vi "foucault control panel.vi"() -> ()   [LabVIEW 2017]
uses:
  typedefs/gain setting.ctl
  typedefs/commandType.ctl
  <vilib>/Analysis/baseanly.llb/Mean (DBL).vi
  popup panels/control panel globals.vi
  <vilib>/Analysis/NI_AALBase.lvlib
panel:
  out "orbit for display":T1 {"height" format="%.1f"; "y offset" format="%.1f"; "x offset" format="%.1f"; "mag  tilt (d)" format="%.1f"; "ax angle (d)" format="%.1f"; "minor axis" format="%.1f"; "maj axis" format="%.1f"}
  out "working magnetomters":bool[](array[boolean])
  out "pulse energy (uJ)":dbl
  out "pulse charge (mC)":sgl
  in  "pulse coil":bool
  in  "zero voltage":bool
  out "predicted precession (deg/hr)":dbl format="%.1f"
  out "minor axis (mm)":dbl format="%.1f"
  in  "bob mass (g)":dbl=550.0
  out "amplitude (mm)":dbl format="%.1f"
  in  "take snapshot":bool
  in  "reset auto coil on pico":bool
  in  "zero field":bool
  in  "num readings\n to average":i32=100 min=1 step=1
  out "gain":dbl
  in  "visible":bool[](array[boolean])=[FALSE, FALSE, FALSE, FALSE, FALSE, FALSE]
  out "pop-up panels":string[](array[string])
  in  "autoscale mag":bool=TRUE
  out "re-synch":bool
  in  "toggle led automatically?":enum16{"NEVER", "WITH COIL", "HALF CYCLE"}(ring)
  out "mag field":cluster{"x":dbl, "y":dbl, "z":dbl}
  out "orbit is":enum16{"clockwise", "counterclockwise"}(ring)
  in  "Freeze Display":bool
  in  "mag type":enum16{"absolute", "relative", "positional"}(ring)
  out "L (m)":dbl
  in  "Display type":enum16{"rolling", "triggered"}(ring)
  in  "Trigger direction":enum16{"falling edge", "rising edge"}(ring)=enum."rising edge"
  out "firmware version":dbl
  in  "auto coil":bool
  in  "pulse duration (ms)":dbl=5.0 format="%#_6f"
  in  "pulse phase (deg)":dbl=40.0 format="%#_6p"
  in  "Gain setting":T2=enum."16.25"
  in  "LED level":u8(slide) scale=0.0..255.0
  in  "manual coil activation":bool
  out "Period":dbl
  in  "hysteresis":dbl=0.05 format="%.3f"
  out "magnet":cluster{dbl[], "Best Linear Fit":dbl[]}[](graph)
  in  "time range (s)":dbl=3.0 format="%#_13g"
  out "voltage":cluster{dbl[], dbl[]}[](graph)
  out "error out":errorcluster
  in  "stop program":bool
  out "VISA resource name":refnum<visa-resource-name>
  # "Update date: 9/28/2022\n(Lab 2 - Fall 2022)"
types:
  T1 = cluster{"maj axis":dbl, "minor axis":dbl, "ax angle (d)":dbl, "mag  tilt (d)":dbl, "x offset":dbl, "y offset":dbl, "height ":dbl}
  T2 = typedef "gain setting.ctl" = enum16{"7.87", "16.25", "30.5", "58.7", "120.6", "238.6", "477.3", "954.6"}
  T3 = typedef "queue cluster.ctl" = cluster{"voltage":T4, "coil":T4, "mag":refnum<queue>, "accel":T4, "crossing":T4, "orbit fit":refnum<queue>, "pulse":T4, "mag0":T4, "fitLocation":refnum<queue>}
  T4 = typedef "reading queue.ctl" = refnum<queue>
  T5 = typedef "reading.ctl" = cluster{"reading type":T6, "time":fxp<+,48,48>, "x":sgl, "y":sgl, "z":sgl, "XSUM":u8}
  T6 = typedef "readingType.ctl" = enum8{"SYNC", "DETVAL", "COILI", "MAGVEC", "ACCVEC", "CROSSING", "MAGVEC0", "MAGVEC1", "MAGVEC2", "MAGVEC3", "MAGVEC4", "MAGVEC5", "MAGVEC6", "MAGVEC7"}
  T7 = typedef "crossing stats.ctl" = cluster{"recent crossing":dbl, "prev crossing":dbl, "crossing-2":dbl, "number of crossings":i32, "period":dbl, "new crossing":bool, "new odd crossing":bool, "slope":dbl}
  T8 = cluster{"maj axis":dbl, "minor axis":dbl, "axis angle (deg)":dbl, "magnet tilt (deg)":dbl, "x offset":dbl, "y offset":dbl, "height above sensor":dbl}
  T9 = enum16{"absolute", "relative", "positional", "position only"}
  T10 = cluster{"pulse energy (uJ)":sgl, "pulse phase":dbl, "v":dbl, "I dt":dbl, "pulse time":dbl, "timing error":dbl}
  T11 = enum32{"Invalid", "Standard", "Closed", "Hidden", "Minimized", "Maximized"}
  T12 = cluster{" xrange":cluster{dbl, dbl}, "yrange":cluster{dbl, dbl}}
  T13 = cluster{"Best Linear Fit":dbl[], "Best Linear Fit":dbl[]}[]
  T14 = typedef "commandType.ctl" = enum16{"G - set gain", "C - activate coil", "D - deactivate coil", "L - set LED", "A - set AUTO", "V - set verbose", "T - set transmission", "R - get version", "Z - zero accelerometer", "F - set auto-flash led", "X - synchronize serial", "Q - reset queues and timers", "S - save configuration"}
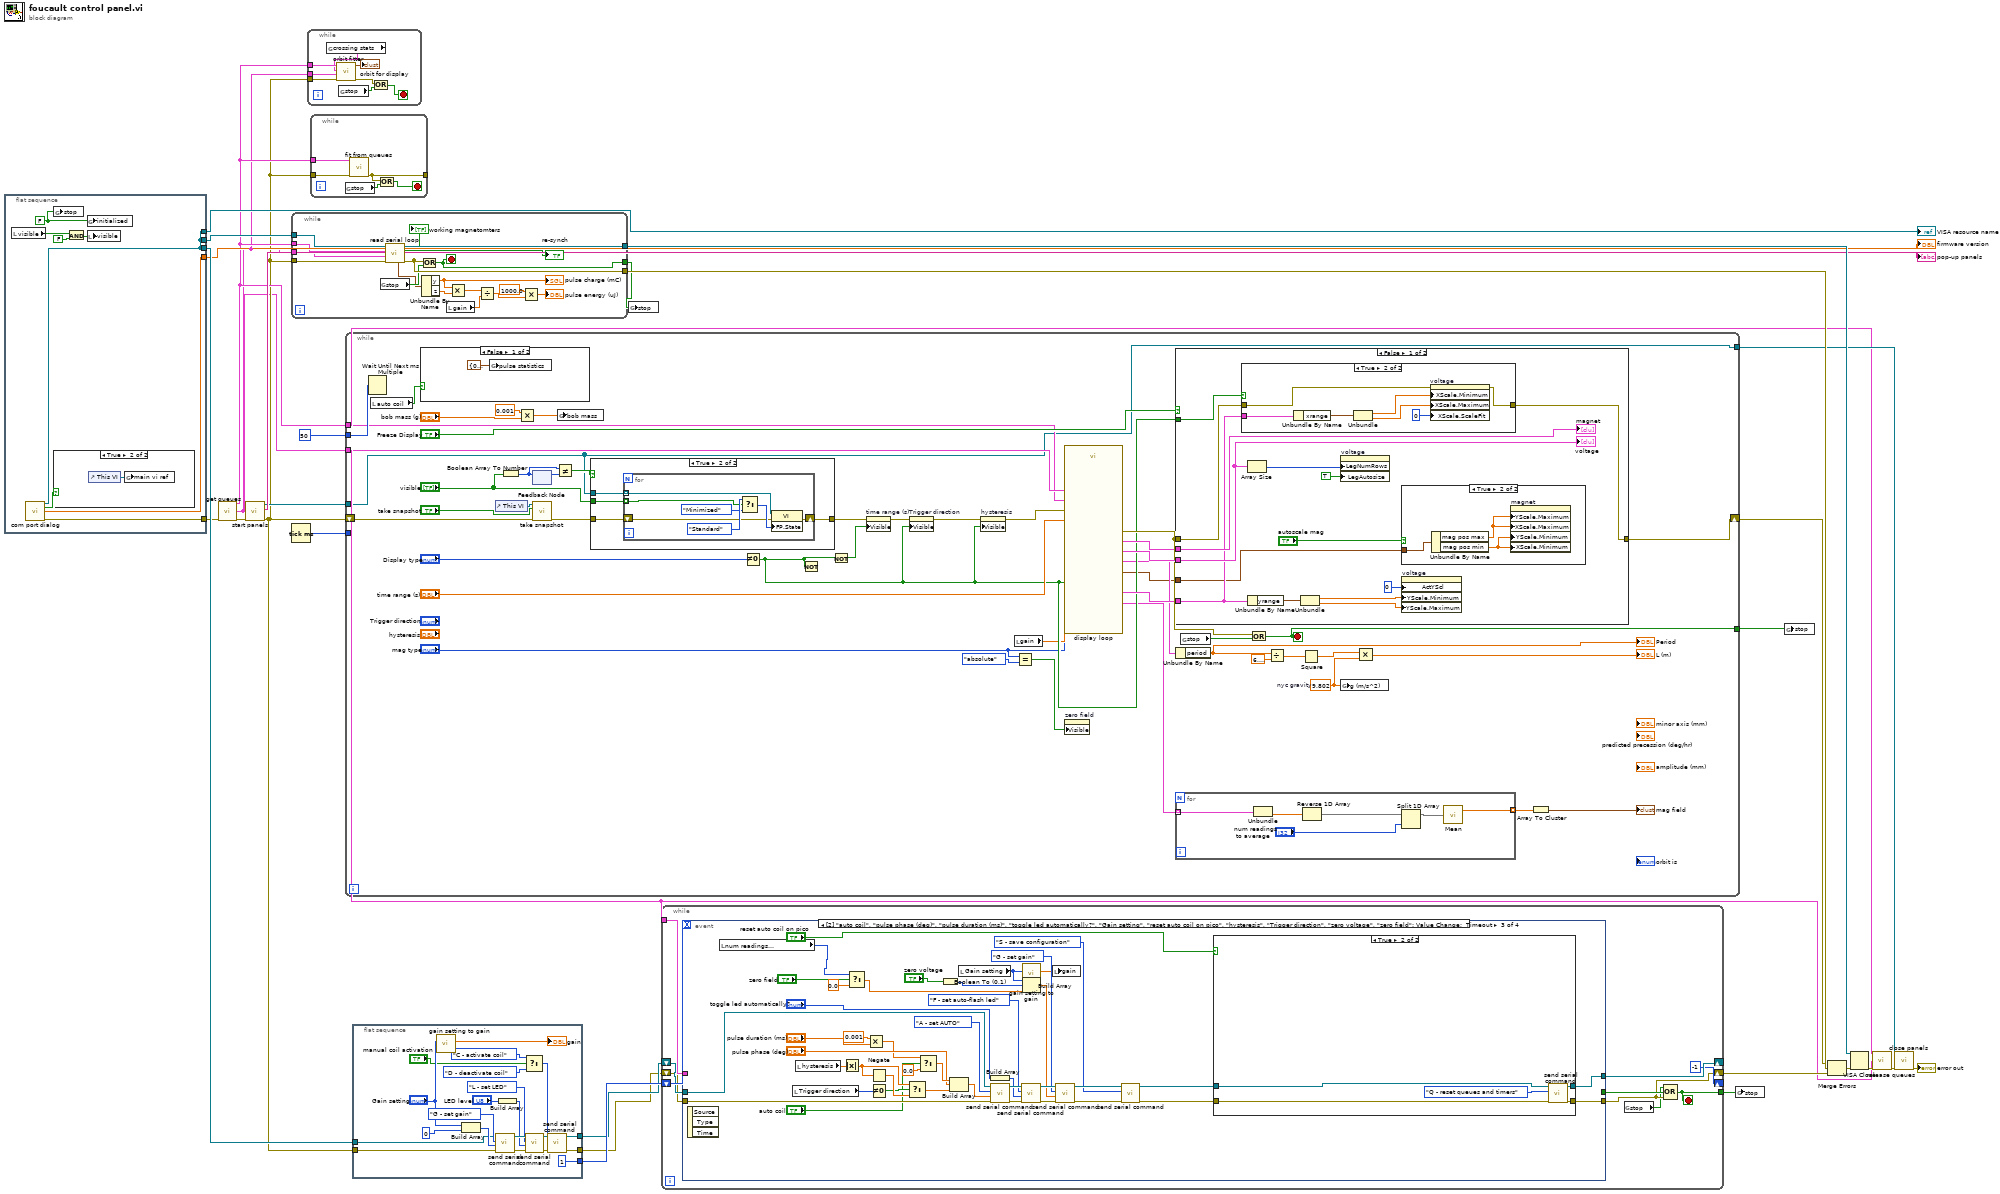
[diagram p0: block diagram]
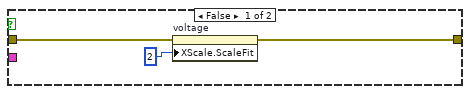
[diagram p5: hidden frame]
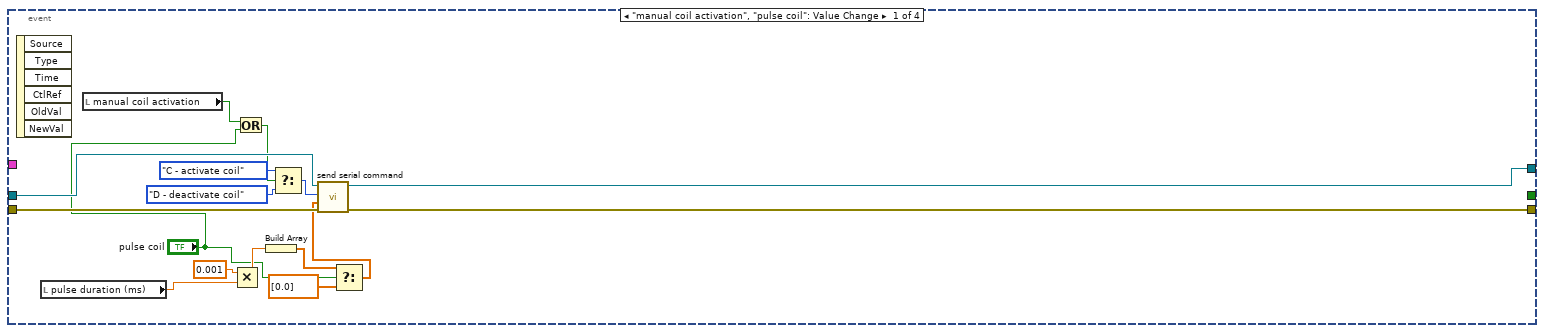
[diagram p7: hidden frame]
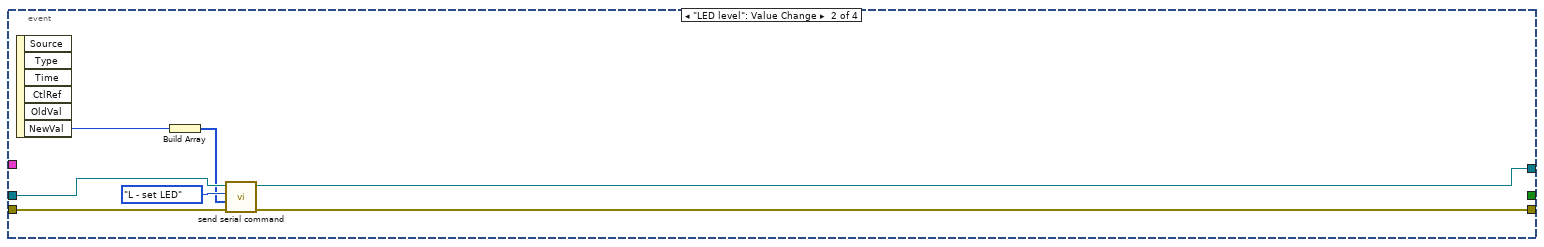
[diagram p8: hidden frame]
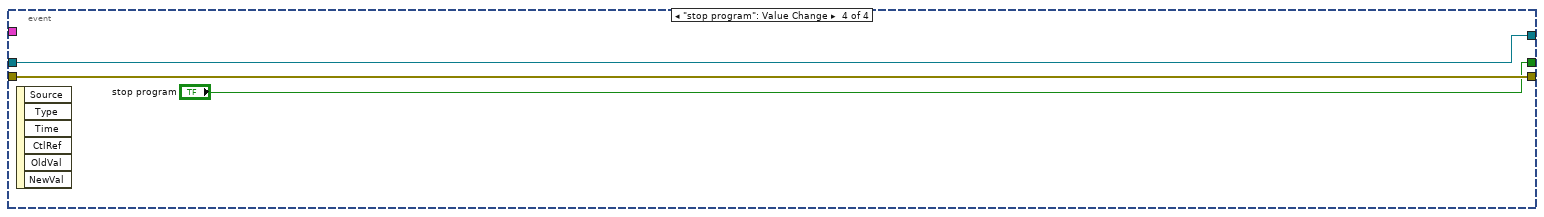
[diagram p10: hidden frame]
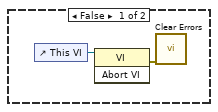
[diagram p11: hidden frame]
diagram:
  n1 = flat-sequence {
    tunnel: [w36] -> w22
    tunnel: [w36] -> w21
    tunnel: [w36] -> w20
    tunnel: [w34] -> w19
    tunnel: [w35] -> w18
    frame #0 {
      w32 = FALSE ("stop 2")
      n2 = local read "visible"() -> (w31:bool[])
      n3 = call "com port dialog.vi"() -> ("VISA resource name out"=w36:refnum<visa-resource-name>, "port opened"=w33:bool, "version"=w34:dbl, "error out"=w35:errorcluster)  [unwired: 11 in, 1 out]
      n4 = global write "control panel globals.vi" "stop"(w32) -> ()
      n5 = case shown="True" w33 {
        frame False {
          n6 = control-ref of="This VI"() -> (w38:refnum<vi>)
          n7 = invoke class="VI" method="Abort VI"(reference=w38) -> (error out=w37:errorcluster)  [unwired: 2 in, 2 out]
          n8 = call <vilib>:"Clear Errors.vi"("error in (no error)"=w37) -> ()  [unwired: 5 in, 2 out]
        }
        frame True {
          n9 = control-ref of="This VI"() -> (w39:refnum<vi>)
          n10 = global write "control panel globals.vi" "main vi ref"(w39) -> ()
        }
      }
      n11 = And(x=w31, y=FALSE) -> (x .and. y?=w29:bool[])
      n12 = global write "control panel globals.vi" "initialized"(w32) -> ()
      n13 = local write "visible"(w29) -> ()
    }
  }
  n14 = call "get queues.vi"("error in (no error)"=w18) -> ("display queues"=w3:T3, "disk queues"=w1:T3, "error out"=w14:errorcluster)  [unwired: 12 in]
  n15 = call "start panels.vi"("error in"=w14) -> ("error out"=w2:errorcluster, "vi names"=→"pop-up panels":string[], "vi refs"=w12:refnum<vi>[])  [unwired: 8 in]
  n16 = while {
    tunnel: w2 -> [w57]
    tunnel: w3 -> [w56]
    tunnel: w1 -> [w55]
    tunnel: [w54] -> w28
    tunnel: [w53] -> w27
    tunnel: [w52] -> w11
    tunnel: w21 -> [w51]
    stop <- w52 stop-if-true
    n17 = global read "control panel globals.vi" "stop"() -> (w49:bool)
    n18 = call "read serial loop.vi"("error in (no error)"=w57, "disk queues"=w55, "display queues"=w56, "serial port"=w51) -> ("error out"=w53:errorcluster, "re-synch"=→"re-synch":bool, "VISA resource name out"=w54:refnum<visa-resource-name>, "last pulse"=w48:T5, "mag set working out"=→"working magnetomters":bool[])  [unwired: 2 in, 1 out]
    n19 = Or(x=w53, y=w49) -> (x .or. y?=w52:bool)
    n20 = Unbundle By Name(w48) -> ("y"=w47:sgl, "z"=w46:sgl)
    "pulse charge (mC)" <- w47
    n21 = local read "gain"() -> (w44:dbl)
    n22 = Multiply(x=w47, y=w46) -> (x*y=w45:sgl)
    n23 = Divide(x=w45, y=w44) -> (x/y=w43:dbl)
    n24 = Multiply(x=1000.0, y=w43) -> (x*y=→"pulse energy (uJ)":dbl)
  }
  n25 = Tick Count (ms)() -> (millisecond timer value=w26:u32)
  n26 = while {
    tunnel: w3 -> [w65]
    tunnel: w2 -> [w61]
    tunnel: w1 -> [w58]
    stop <- w62 stop-if-true
    n27 = global read "control panel globals.vi" "crossing stats"() -> (w60:T7)
    n28 = call "orbit fitter.vi"("error in (no error)"=w61, "disk queues"=w58, "crossing stats"=w60, "display queues"=w65) -> ("error out"=w64:errorcluster, "orbit for display"=→"orbit for display":T8)  [unwired: 6 in]
    n29 = global read "control panel globals.vi" "stop"() -> (w63:bool)
    n30 = Or(x=w64, y=w63) -> (x .or. y?=w62:bool)
  }
  n31 = while {
    tunnel: w3 -> [w70]
    tunnel: w2 -> [w69]
    tunnel: [w68] -> _
    stop <- w66 stop-if-true
    n32 = global read "control panel globals.vi" "stop"() -> (w67:bool)
    n33 = call "fit from queues.vi"("error in (no error)"=w69, "display queues"=w70) -> ("error out"=w68:errorcluster)  [unwired: 9 in]
    n34 = Or(x=w68, y=w67) -> (x .or. y?=w66:bool)
  }
  n35 = while {
    tunnel: w26 -> [_]
    shift-right: [w103] -> w15
    shift-left: w2 -> [w82]
    tunnel: w3 -> [w93]
    tunnel: [w116] -> w9
    tunnel: w1 -> [w109]
    tunnel: i64 50 ("update (ms)") -> [w108]
    tunnel: w12 -> [w83]
    tunnel: [w83] -> w6
    stop <- w116 stop-if-true
    w77 = 9.802  # nyc gravity
    n36 = Wait Until Next ms Multiple(millisecond multiple=w108) -> ()  [unwired: 1 out]
    n37 = local read "auto coil"() -> (w76:bool)
    n38 = case shown="False" w76 {
      frame False {
        n39 = global write "control panel globals.vi" "pulse statistics"(T10 {"pulse energy (uJ)"=0.0, "pulse phase"=0.0, "v"=0.0, "I dt"=0.0, "pulse time"=0.0, "timing error"=0.0} ("pulse statistics")) -> ()
      }
      frame True {
      }
    }
    n40 = control-ref of="This VI"() -> (w80:refnum<vi>)
    n41 = Boolean Array To Number(Boolean array="visible") -> (number=w89:u32)
    n42 = Multiply(x=0.001, y="bob mass (g)") -> (x*y=w74:dbl)
    n43 = feedback-in #1(w89) -> ()
    n44 = feedback #1() -> (w88:u32)  [unwired: 1 in]
    n45 = call "take snapshot.vi"("error in (no error)"=w82, "take snapshot"="take snapshot", "vi ref"=w80) -> ("error out"=w81:errorcluster)  [unwired: 8 in]
    n46 = Not Equal?(x=w89, y=w88) -> (x != y?=w87:bool)
    n47 = global write "control panel globals.vi" "bob mass"(w74) -> ()
    n48 = case shown="True" w87 {
      tunnel: w83 -> [_ w123]
      tunnel: w81 -> [w119 w122]
      tunnel: [w119 w121] -> w92
      tunnel: "visible" -> [_ w120]
      frame False {
      }
      frame True {
        n49 = for {
          tunnel: w123 -> [w130] mode=indexing
          shift-right: [w125] -> w121
          shift-left: w122 -> [w126]
          tunnel: w120 -> [w124] mode=indexing
          n50 = Select(t=T11."Standard" ("Front Panel Window:State"), s=w124, f=T11."Minimized") -> (s? t:f=w127:T11)
          n51 = property class="VI"(reference=w130, error in=w126, "FP.State"=w127) -> (error out=w125:errorcluster)  [unwired: 1 out]
        }
      }
    }
    n52 = Not Equal To 0?(x="Display type") -> (x != 0?=w98:bool)
    n53 = Not(x=w98) -> ()  [unwired: 1 out]
    n54 = Not(x=w98) -> (.not. x?=w111:bool)
    n55 = property on="time range (s)" class="DigNum (strict)"(error in=w92, "Visible"=w111) -> (error out=w114:errorcluster)  [unwired: 1 in, 1 out]
    n56 = property on="Trigger direction" class="Enum (strict)"(error in=w114, "Visible"=w98) -> (error out=w113:errorcluster)  [unwired: 1 in, 1 out]
    n57 = property on="hysteresis" class="DigNum (strict)"(error in=w113, "Visible"=w98) -> (error out=w112:errorcluster)  [unwired: 1 in, 1 out]
    n58 = local read "gain"() -> (w97:dbl)
    n59 = Equal?(x="mag type", y=T9."absolute") -> (x = y?=w84:bool)
    n60 = call "display loop.vi"("display queues"=w93, "time range (s)"="time range (s)", "mag type"="mag type", "error in"=w112, "trigger"=w98, "disk queues"=w109, "gain"=w97) -> ("magnet vs time"=w78:cluster{dbl[], dbl[]}[], "mag pos axes limits"=w94:cluster{"mag pos max":dbl, "mag pos min":dbl}, "voltage axes"=w104:T12, "crossing stats"=w96:T7, "voltage graphs"=w107:cluster{dbl[], dbl[]}[], "magnet graphs"=w101:T13, "error out"=w105:errorcluster)  [unwired: 14 in]
    n61 = property on="zero field" class="Bool"("Visible"=w84) -> ()  [unwired: 2 in, 2 out]
    n62 = case shown="False" "Freeze Display" {
      tunnel: w98 -> [w150 _]
      tunnel: w105 -> [w149 w164]
      tunnel: w104 -> [w141 _]
      tunnel: [w148 w164] -> w103
      tunnel: w107 -> [w146 _]
      tunnel: w101 -> [w143 _]
      tunnel: w94 -> [w137 _]
      frame False {
        n63 = case shown="True" w150 {
          tunnel: w149 -> [w156 w163]
          tunnel: w141 -> [_ w160]
          tunnel: [w154 w162] -> w148
          frame False {
            n64 = property on="voltage" class="XYGraph (strict)"(error in=w156, "XScale.ScaleFit"=u8 2 ("X Scale.Scale Fit")) -> (error out=w154:errorcluster)  [unwired: 1 in, 1 out]
          }
          frame True {
            n65 = Unbundle By Name(w160) -> ("xrange"=w159:cluster{dbl, dbl})
            n66 = Unbundle(w159) -> (w158:dbl, w157:dbl)
            n67 = property on="voltage" class="XYGraph (strict)"(error in=w163, "XScale.Minimum"=w158, "XScale.Maximum"=w157, "XScale.ScaleFit"=u8 0 ("X Scale.Scale Fit")) -> (error out=w162:errorcluster)  [unwired: 1 in, 1 out]
          }
        }
        n68 = Array Size(array=w146) -> (size(s)=w145:i32)
        n69 = Unbundle By Name(w141) -> ("yrange"=w140:cluster{dbl, dbl})
        n70 = Unbundle(w140) -> (w139:dbl, w138:dbl)
        n71 = property on="voltage" class="XYGraph (strict)"("LegNumRows"=w145, "LegAutosize"=TRUE ("Legend:Autosize")) -> ()  [unwired: 2 in, 2 out]
        n72 = case shown="True" "autoscale mag" {
          tunnel: w137 -> [_ w153]
          frame False {
          }
          frame True {
            n73 = Unbundle By Name(w153) -> ("mag pos max"=w152:dbl, "mag pos min"=w151:dbl)
            n74 = property on="magnet" class="XYGraph (strict)"("YScale.Maximum"=w152, "XScale.Maximum"=w152, "YScale.Minimum"=w151, "XScale.Minimum"=w151) -> ()  [unwired: 2 in, 2 out]
          }
        }
        n75 = property on="voltage" class="XYGraph (strict)"("ActYScl"=0 ("Active Y Scale"), "YScale.Minimum"=w139, "YScale.Maximum"=w138) -> ()  [unwired: 2 in, 2 out]
        "voltage" <- w146
        "magnet" <- w143
      }
      frame True {
      }
    }
    n76 = Unbundle By Name(w96) -> ("period"=w95:dbl)
    "Period" <- w95
    n77 = for {
      tunnel: w78 -> [w136] mode=indexing
      tunnel: [w131] -> w100 mode=indexing
      n78 = Unbundle(w136) -> (w135:dbl[])  [unwired: 1 out]
      n79 = Reverse 1D Array(array=w135) -> (reversed array=w134:dbl[])
      n80 = Split 1D Array(array=w134, index="num readings\n to average") -> (first subarray=w132:dbl[])  [unwired: 1 out]
      n81 = call-poly <vilib>:"Mean.vi"("X"=w132) -> ("mean"=w131:dbl)  [unwired: 1 out]
    }
    n82 = global read "control panel globals.vi" "stop"() -> (w91:bool)
    n83 = Or(x=w105, y=w91) -> (x .or. y?=w116:bool)
    n84 = Divide(x=w95, y=6.283185307179586) -> (x/y=w72:dbl)
    n85 = Square(x=w72) -> (x^2=w110:dbl)
    n86 = global write "control panel globals.vi" "g (m/s^2)"(w77) -> ()
    n87 = Multiply(x=w110, y=w77) -> (x*y=→"L (m)":dbl)
    n88 = Array To Cluster(array=w100) -> (cluster=→"mag field":cluster{"[0]":dbl, "[1]":dbl, "[2]":dbl})
  }
  n89 = flat-sequence {
    tunnel: [w166] -> w5
    tunnel: [w167] -> w4
    tunnel: [1] -> w25
    tunnel: w2 -> [w170]
    tunnel: w20 -> [w169]
    frame #0 {
      n90 = call "gain setting to gain.vi"("Gain setting"="Gain setting") -> ("gain"=→"gain":dbl)  [unwired: 10 in]
      n91 = Build Array("Gain setting", 0) -> (w180:i32[])
      n92 = call "send serial command.vi"("error in (no error)"=w170, "data"=w180, "Command"=commandType."G - set gain", "visa resource"=w169) -> ("error out"=w185:errorcluster, "VISA resource name out"=w184:refnum<visa-resource-name>)  [unwired: 5 in, 1 out]
      n93 = Build Array("LED level") -> (w177:u8[])
      n94 = Select(t=commandType."C - activate coil" ("Command"), s="manual coil activation", f=commandType."D - deactivate coil") -> (s? t:f=w172:T14)
      n95 = call "send serial command.vi"("error in (no error)"=w185, "data"=w177, "Command"=commandType."L - set LED", "visa resource"=w184) -> ("error out"=w182:errorcluster, "VISA resource name out"=w183:refnum<visa-resource-name>)  [unwired: 5 in, 1 out]
      n96 = call "send serial command.vi"("error in (no error)"=w182, "Command"=w172, "visa resource"=w183) -> ("error out"=w167:errorcluster, "VISA resource name out"=w166:refnum<visa-resource-name>)  [unwired: 6 in, 1 out]
    }
  }
  n97 = global write "control panel globals.vi" "stop"(w11) -> ()
  n98 = while {
    shift-right: [w194] -> _
    shift-left: w5 -> [w187]
    shift-right: [w191] -> w23
    shift-left: w4 -> [w186]
    shift-right: [-1] -> _
    shift-left: w25 -> [w195]
    tunnel: [w190] -> w10
    tunnel: w1 -> [w189]
    stop <- w190 stop-if-true
    n99 = event shown="[2] \"auto coil\", \"pulse phase (deg)\", \"pulse duration (ms)\", \"toggle led automatically?\", \"Gain setting\", \"reset auto coil on pico\", \"hysteresis\", \"Trigger direction\", \"zero voltage\", \"zero field\": Value Change;  Timeout" {
      selector: _ -> [_ _ _ _]
      dyn-events: _ -> [_ _ _ _]
      timeout: w195 -> [_ _ _ _]
      tunnel: w187 -> [w211 w218 w260 w269]
      tunnel: w186 -> [w210 w216 w258 w270]
      tunnel: [w209 w215 w227 w269] -> w194
      tunnel: [w208 w214 w226 w270] -> w191
      tunnel: [_ _ _ "stop program"] -> w192
      tunnel: w189 -> [_ _ _ _]
      event "manual coil activation", "pulse coil": Value Change {
        n100 = event-data() -> ()  [unwired: 1 in, 6 out]
        n101 = local read "pulse duration (ms)"() -> (w201:dbl)
        n102 = local read "manual coil activation"() -> (w204:bool)
        n103 = Multiply(x=0.001, y=w201) -> (x*y=w200:dbl)
        n104 = Or(x=w204, y="pulse coil") -> (x .or. y?=w203:bool)
        n105 = Build Array(w200) -> (w199:dbl[])
        n106 = Select(t=commandType."C - activate coil" ("Command"), s=w203, f=commandType."D - deactivate coil") -> (s? t:f=w205:T14)
        n107 = Select(t=w199, s="pulse coil", f=dbl[] [0.0]) -> (s? t:f=w196:dbl[])
        n108 = call "send serial command.vi"("error in (no error)"=w210, "data"=w196, "Command"=w205, "visa resource"=w211) -> ("error out"=w208:errorcluster, "VISA resource name out"=w209:refnum<visa-resource-name>)  [unwired: 5 in, 1 out]
      }
      event "LED level": Value Change {
        n109 = event-data() -> ("NewVal"=w213:u8)  [unwired: 1 in, 5 out]
        n110 = Build Array(w213) -> (w212:u8[])
        n111 = call "send serial command.vi"("error in (no error)"=w216, "data"=w212, "Command"=commandType."L - set LED", "visa resource"=w218) -> ("error out"=w214:errorcluster, "VISA resource name out"=w215:refnum<visa-resource-name>)  [unwired: 5 in, 1 out]
      }
      event "auto coil", "pulse phase (deg)", "pulse duration (ms)", "toggle led automatically?", "reset auto coil on pico", "hysteresis", "Trigger direction", "zero voltage", "zero field": Value Change; Timeout {
        n112 = event-data() -> ()  [unwired: 1 in, 3 out]
        n113 = local read "num readings\n to average"() -> (w219:i32)
        n114 = local read "Trigger direction"() -> (w243:enum16{"falling edge", "rising edge"})
        n115 = local read "hysteresis"() -> (w232:dbl)
        n116 = Absolute Value(x=w232) -> (abs(x)=w255:dbl)
        n117 = Select(t=w219, s="zero field", f=0.0) -> (s? t:f=w220:dbl)
        n118 = Multiply(x=0.001, y="pulse duration (ms)") -> (x*y=w250:dbl)
        n119 = Negate(x=w255) -> (-x=w254:dbl)
        n120 = Not Equal To 0?(x=w243) -> (x != 0?=w242:bool)
        n121 = Select(t=w255, s=w242, f=w254) -> (s? t:f=w231:dbl)
        n122 = Select(t=w250, s="auto coil", f=0.0) -> (s? t:f=w253:dbl)
        n123 = Boolean To (0,1)(Boolean="zero voltage") -> (0, 1=w223:i16)
        n124 = Build Array(w253, "pulse phase (deg)", w231) -> (w251:dbl[])
        n125 = local read "Gain setting"() -> (w234:T2)
        n126 = Build Array("toggle led automatically?") -> (w244:enum16{"NEVER", "WITH COIL", "HALF CYCLE"}[])
        n127 = call "send serial command.vi"("error in (no error)"=w258, "data"=w251, "Command"=commandType."A - set AUTO", "visa resource"=w260) -> ("error out"=w247:errorcluster, "VISA resource name out"=w248:refnum<visa-resource-name>)  [unwired: 5 in, 1 out]
        n128 = call "send serial command.vi"("error in (no error)"=w247, "data"=w244, "Command"=commandType."F - set auto-flash led", "visa resource"=w248) -> ("error out"=w241:errorcluster, "VISA resource name out"=w240:refnum<visa-resource-name>)  [unwired: 5 in, 1 out]
        n129 = call "gain setting to gain.vi"("Gain setting"=w234) -> ("gain"=w233:dbl)  [unwired: 10 in]
        n130 = Build Array(w234, w223, w220) -> (w238:dbl[])
        n131 = local write "gain"(w233) -> ()
        n132 = call "send serial command.vi"("error in (no error)"=w241, "data"=w238, "Command"=commandType."G - set gain", "visa resource"=w240) -> ("error out"=w237:errorcluster, "VISA resource name out"=w236:refnum<visa-resource-name>)  [unwired: 5 in, 1 out]
        n133 = call "send serial command.vi"("error in (no error)"=w237, "Command"=commandType."S - save configuration", "visa resource"=w236) -> ("error out"=w229:errorcluster, "VISA resource name out"=w230:refnum<visa-resource-name>)  [unwired: 6 in, 1 out]
        n134 = case shown="True" "reset auto coil on pico" {
          tunnel: w230 -> [w262 w267]
          tunnel: w229 -> [w261 w266]
          tunnel: [w262 w264] -> w227
          tunnel: [w261 w263] -> w226
          frame False {
          }
          frame True {
            n135 = call "send serial command.vi"("error in (no error)"=w266, "Command"=commandType."Q - reset queues and timers", "visa resource"=w267) -> ("error out"=w263:errorcluster, "VISA resource name out"=w264:refnum<visa-resource-name>)  [unwired: 6 in, 1 out]
          }
        }
      }
      event "stop program": Value Change {
        n136 = event-data() -> ()  [unwired: 1 in, 6 out]
      }
    }
    n137 = global read "control panel globals.vi" "stop"() -> (w188:bool)
    n138 = Compound Arithmetic op=OR(w188, w192, w191) -> (w190:bool)
  }
  n139 = global write "control panel globals.vi" "stop"(w10) -> ()
  n140 = global write "control panel globals.vi" "stop"(w9) -> ()
  n141 = Merge Errors(w15, w27, w23) -> (w24:errorcluster)
  n142 = VISA Close(VISA resource name=w28, error in (no error)=w24) -> (error out=w17:errorcluster)
  n143 = call "release queues.vi"("display queues"=w3, "disk queues"=w1, "error in (no error)"=w17) -> ("error out"=w8:errorcluster)  [unwired: 12 in]
  n144 = call "close panels.vi"("error in"=w8, "vi refs"=w6) -> ("error out"=→"error out":errorcluster)  [unwired: 9 in]
  "firmware version" <- w19
  "VISA resource name" <- w22
